vi "UpdateDisplay.vi"(10 "Channel":i32, 11 "Array":waveform(dbl)[](array[waveform])) -> (3 "Image":T1(plugin-control))   [LabVIEW 2012]
uses:
  <vilib>/picture/picture.llb/imagedata.ctl
  <vilib>/Analysis/baseanly.llb/Mean (DBL).vi
  <vilib>/Analysis/NI_AALBase.lvlib
panel:
  in  "Numeric":dbl
  out "Waveform Chart":dbl(graph)
  in  "Downsample":i32=4
  out "Pixel count":i32
  in  "offset":i32
  in  "Gain":dbl=5000.0
  in  "width":i32=300
  in  "height":i32=300
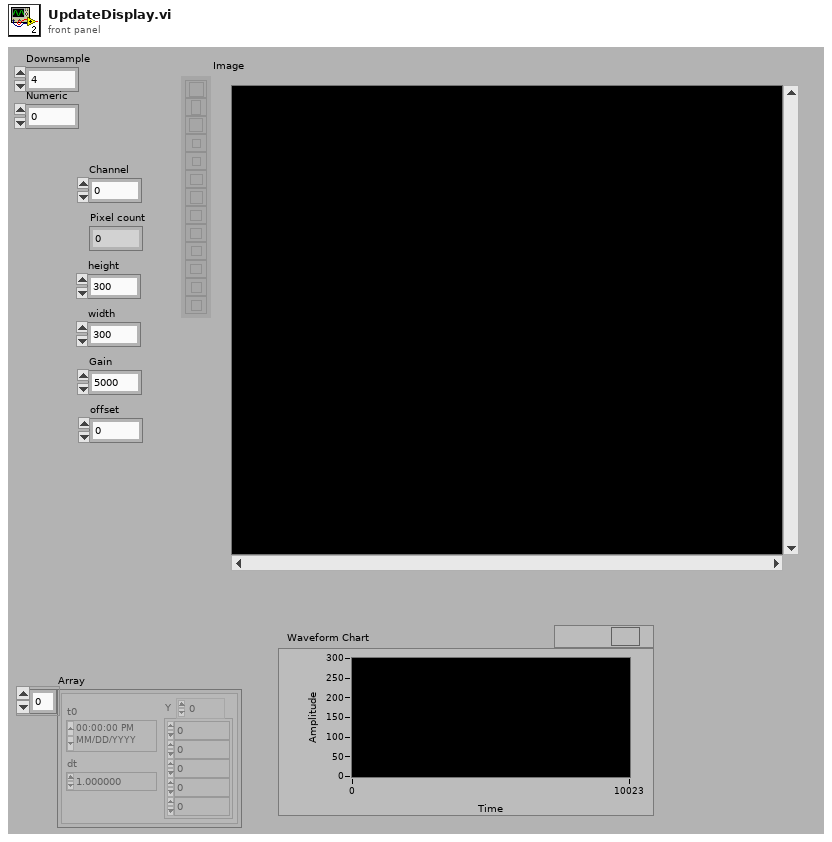
[diagram p1: front panel]
types:
  T1 = typedef "IMAQ Image.ctl" = refnum<image>
  T2 = typedef "imagedata.ctl" = cluster{"image type":i32, "image depth":i32, "image":u8[], "mask":u8[], "colors":u32[], "Rectangle":cluster{"left":i16, "top":i16, "right":i16, "bottom":i16}}
  T3 = typedef "Image Type" = u32
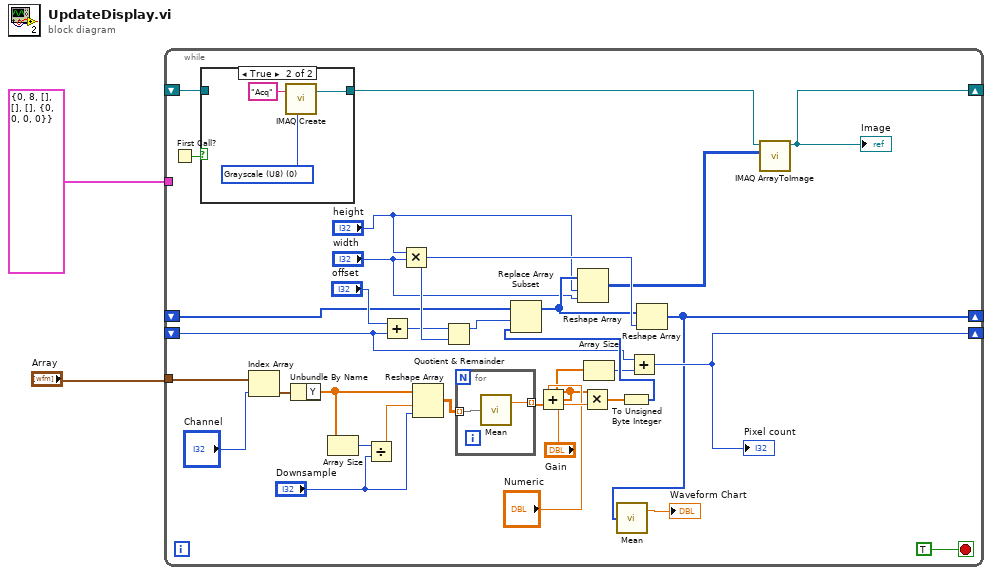
[diagram p0: block diagram]
diagram:
  n1 = while {
    tunnel: "Array" -> [w24]
    shift-right: [w23] -> _
    shift-left: _ -> [w21]
    shift-right: [w6] -> _
    shift-left: _ -> [w22]
    tunnel: T2 {"image type"=0, "image depth"=8, "image"=[], "mask"=[], "colors"=[], "Rectangle"={"left"=0, "top"=0, "right"=0, "bottom"=0}} ("image data") -> [_]
    shift-right: [w9] -> _
    shift-left: _ -> [w15]
    stop <- TRUE stop-if-true
    n2 = First Call?() -> (First Call?: T/F=w14:bool)
    n3 = case shown="True" w14 {
      tunnel: [w36 w38] -> w13
      tunnel: w15 -> [w36 _]
      frame False {
      }
      frame True {
        w37 = T3 0 items=["Grayscale (U8)", "Grayscale (I16)", "Grayscale (SGL)", "Complex (CSG)", "RGB (U32)", "HSL (U32)", "RGB (U64)", "Grayscale (U16)"] ("Image Type")
        n4 = call "IMAQ Create"("Image Name"="Acq", "Image Type"=w37) -> ("New Image"=w38:T1)  [unwired: 2 in, 2 out]
      }
    }
    n5 = Index Array(array=w24, index="Channel") -> (element=w26:waveform(dbl))
    n6 = Unbundle By Name(w26) -> ("Y"=w20:dbl[])
    n7 = Array Size(array=w20) -> (size(s)=w19:i32)
    n8 = Divide(x=w19, y="Downsample") -> (x/y=w18:dbl)
    n9 = Add(x="offset", y=w21) -> (x+y=w32:i32)
    n10 = Multiply(x="height", y="width") -> (x*y=w34:i32)
    n11 = Reshape Array(w20, w18, "Downsample") -> (w16:dbl[][])
    n12 = Quotient & Remainder(x=w32, y=w34) -> (x-y*floor(x/y)=w33:i32)  [unwired: 1 out]
    n13 = for {
      tunnel: w16 -> [w41] mode=indexing
      tunnel: [w40] -> w5 mode=indexing
      n14 = call-poly <vilib>:"Mean.vi"("X"=w41) -> ("mean"=w40:dbl)  [unwired: 1 out]
    }
    n15 = Add(x="Numeric", y=w5) -> (x+y=w3:dbl[])
    n16 = Multiply(x=w3, y="Gain") -> (x*y=w29:dbl[])
    n17 = Array Size(array=w3) -> (size(s)=w27:i32)
    n18 = To Unsigned Byte Integer(number=w29) -> (unsigned 8bit integer=w30:u8[])
    n19 = Replace Array Subset(array=w22, new element=w30, index=w33) -> (w12:u8[])
    n20 = Reshape Array(w12, "height", "width") -> (w8:u8[][])
    n21 = Add(x=w21, y=w27) -> (x+y=w23:i32)
    "Pixel count" <- w23
    n22 = Reshape Array(w12, w34) -> (w6:u8[])
    n23 = call-poly <vilib>:"Mean.vi"("X"=w6) -> ("mean"=→"Waveform Chart":dbl)  [unwired: 1 out]
    n24 = call "IMAQ ArrayToImage"("Image Pixels (U8)"=w8, "Image"=w13) -> ("Image Out"=w9:T1)  [unwired: 4 in, 5 out]
    "Image" <- w9
  }
